vi "Example.vi"   [LabVIEW 2016]
uses:
  <vilib>/NXT/Block Support/NXT_InputPort.ctl
  <vilib>/NXT/Hardware/Plugins/Tetrix DC Motor/TetrixDCMotorAddress.ctl
  <vilib>/NXT/Hardware/Plugins/Tetrix 180 deg Servo/Tetrix180ServoAddress.ctl
  <vilib>/NXT/NXTIO Xnodes/NXTIONodeSubVIs/TETRIX IO Move Servos.vi
  <vilib>/NXT/Dual Mode Library/Waits/Wait_Num.vi
  <vilib>/NXT/NXTIO Xnodes/NXTIONodeSubVIs/TETRIX IO Move DC Motors.vi
  <vilib>/NXT/Dual Mode Library/Waits/Wait_EV3_Ultrasonic_Centimeter_Closer.vi
  <vilib>/NXT/NXTIO Xnodes/NXTIONodeSubVIs/TETRIX IO Stop DC Motors.vi
  <vilib>/NXT/NXTIO Xnodes/AddressXNode/NXTIOAddress.xnode
  Test.lvrbt
  <vilib>/NXT/Subs/LVHSConnector.ctl
  <vilib>/NXT/NXTIO Xnodes/NXTIOXNode/NXTIO.xnode
  <vilib>/NXT/LegoClasses/BrickReference/BrickReference.lvclass
types:
  T1 = typedef "NXT_InputPort.ctl" = u32
  T2 = typedef "Tetrix180ServoAddress.ctl" = i32
  T3 = cluster{"Tetrix180Servo":T2, "Tetrix180Servo":T2, "Tetrix180Servo":T2}
  T4 = typedef "LVHSConnector.ctl" = refnum<class "BrickReference.lvclass">
  T5 = typedef "TetrixDCMotorAddress.ctl" = i32
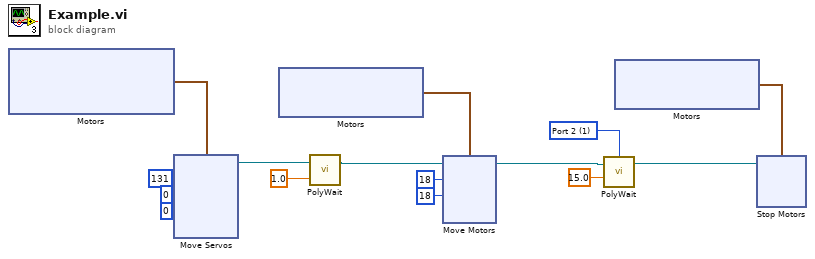
[diagram p0: block diagram]
diagram:
  w3 = T1 1 items=["Port 1", "Port 2", "Port 3", "Port 4"] ("Port (Port 1)")
  n1 = xnode "Motors"() -> ("Motor"=w12:T3)
  n2 = xnode "Move Servos"("Position 3"=u8 0, "Position 2"=u8 0, "Position 1"=u8 131, "Motors"=w12) -> ("NXT/EV3"=w6:T4)  [unwired: 1 in]
  n3 = xnode "Motors"() -> ("Motor"=w15:cluster{"TetrixDCMotor":T5, "TetrixDCMotor":T5})
  n4 = call-poly <vilib>:"PolyWait.vi"("Time (1 sec)"=sgl 1.0, "NXT/EV3"=w6) -> ("NXT/EV3"=w8:T4)  [unwired: 2 in]
  n5 = xnode "Move Motors"("Power/Speed 2"=i8 18, "Power/Speed 1"=i8 18, "Motors"=w15, "NXT/EV3"=w8) -> ("NXT/EV3"=w1:T4)
  n6 = call-poly <vilib>:"PolyWait.vi"("Centimeters (40)"=sgl 15.0, "NXT/EV3"=w1, "Port (Port 1)"=w3) -> ("NXT/EV3"=w4:T4)  [unwired: 1 in]
  n7 = xnode "Motors"() -> ("Motor"=w5:cluster{"TetrixDCMotor":T5, "TetrixDCMotor":T5})
  n8 = xnode "Stop Motors"("Motors"=w5, "NXT/EV3"=w4) -> ()  [unwired: 1 out]
